vi "Auto.vi"() -> ()   [LabVIEW 2020]
uses:
  Global_Variable/Global.vi
  Global_Variable/A180648.vi
  Global_Variable/System_Conf.vi
  Libraries/S7/S7.lvlib
panel:
  out "前序":string
  out "用户事件输出":refnum<user-event>
  out "磨合正向初始化":bool
  out "工位三开始计时1":bool
  out "产品变更_Event":refnum<user-event>
  out "T1+T2":dbl
  out "T2":dbl
  out "T1":dbl
  out "吸收电流":sgl
  out "输出扭矩(大)":sgl
  out "输入扭矩":sgl
  out "力特性逆向去程":bool
  out "力特性正向去程":bool
  out "力特性逆向回程":bool
  out "力特性正向回程":bool
  out "工位三开始计时":bool
  out "工位二开始计时":bool
  out "功能正向初始化":bool
  out "功能逆向初始化":bool
  out "空载逆向初始化":bool
  out "空载正向初始化":bool
  out "试验项目":T1(tab)
  out "拉压曲线":cluster{dbl[], dbl[]}[](graph)
  out "侧铆曲线":cluster{dbl[], dbl[]}[](graph)
  out "0°曲线":cluster{dbl[], dbl[]}[](graph)
  out "45°曲线":cluster{dbl[], dbl[]}[](graph)
  out "力特性试验":cluster{dbl[], dbl[]}[](graph)
  out "功能试验":cluster{dbl[], dbl[]}[](graph)
  out "电流特性试验":cluster{dbl[], dbl[]}[](graph)
  out "逆向空载试验":cluster{dbl[], dbl[]}[](graph)
  out "磨合":cluster{dbl[], dbl[]}[](graph)
  in  "判定结果":bool[][](array[boolean])=[[TRUE]]
  in  "STEP":string
  # "车速0"
  # "车速1"
  # "车速2"
  # "车速3"
  # "车速4"
  # "车速5"
  # "车速0"
  # "车速1"
  # "车速2"
  # "车速3"
  # "车速4"
  # "车速5"
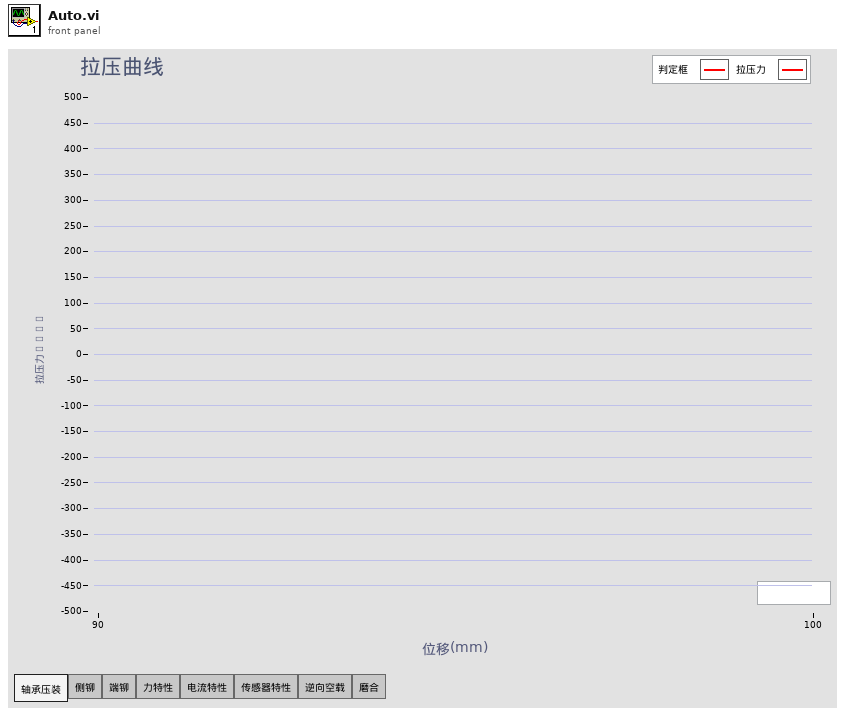
[diagram p1: front panel]
types:
  T1 = enum32{"轴承压装", "侧铆", "端铆", "力特性", "电流特性", "传感器特性", "逆向空载", "磨合"}
  T2 = enum32{"Invalid", "Standard", "Closed", "Hidden", "Minimized", "Maximized"}
  T3 = cluster{"输入轴扭矩":dbl, "输出轴扭矩小量程":dbl, "输出轴扭矩大量程":dbl}
  T4 = typedef "System_conf.ctl" = cluster{"空载滤波":bool, "逆向空载滤波":bool, "空载扭矩系数":dbl, "逆向空载扭矩系数":dbl}
  T5 = cluster{"位移":cluster{"单位":string, "下限":dbl, "上限":dbl}, "拉力":cluster{"单位":string, "下限":dbl, "上限":dbl}, "位移1":cluster{"单位":string, "下限":dbl, "上限":dbl}, "压力":cluster{"单位":string, "下限":dbl, "上限":dbl}}
  T6 = cluster{"拉力最大值":cluster{"单位":string, "下限":dbl, "上限":dbl}, "拉力最小值":cluster{"单位":string, "下限":dbl, "上限":dbl}, "拉力波动":cluster{"单位":string, "下限":dbl, "上限":dbl}, "压力最大值":cluster{"单位":string, "下限":dbl, "上限":dbl}, "压力最小值":cluster{"单位":string, "下限":dbl, "上限":dbl}, "压力波动":cluster{"单位":string, "下限":dbl, "上限":dbl}}
  T7 = cluster{"输入旋转位移":sgl, "电缸":sgl, "工装移载位移":sgl, "345":sgl, "电缸位移":sgl, "打算":sgl, "输出扭矩(大)":sgl, "132":sgl, "拉压力":sgl, "sad":sgl}
  T8 = typedef "lveventtype.ctl" = enum32{"Null", "Timeout", "Annotation Menu Selection", "Annotation Menu Selection?", "App Instance Close", "App Instance Close?", "Autoscale Range Change", "Bookmark Info Change", "Cell Edit", "Cell Edit?", "Cursor Grab", "Cursor Grab?", "Cursor Menu Selection", "Cursor Menu Selection?", "Cursor Move", "Cursor Release", "Data Change", "Direction Change", "Display State Change", "Drag Ended", "Drag Enter", "Drag Leave", "Drag Over", "Drag Source Update", "Drag Starting", "Drag Starting?", "Drop", "Exec State Change", "Key Down", "Key Down?", "Key Repeat", "Key Repeat?", "Key Up", "Listbox Double Click", "Menu Activation?", "Menu Selection (App)", "Menu Selection? (App)", "Menu Selection (User)", "Mouse Down", "Mouse Down?", "Mouse Enter", "Mouse Leave", "Mouse Move", "Mouse Up", "Mouse Wheel", "NI Security User Change (App)", "Pane Size", "Panel Close", "Panel Close?", "Panel Resize", "Plot Attribute Change", "Scale Range Change", "Shortcut Menu Activation?", "Shortcut Menu Selection (App)", "Shortcut Menu Selection? (App)", "Shortcut Menu Selection (User)", "Tree Double Click", "Tree Drag", "Tree Drag?", "Tree Drop", "Tree Drop?", "Tree Item Close", "Tree Item Close?", "Tree Item Open", "Tree Item Open?", "User Event", "Value Change"}
  T9 = typedef "LVPoint32TypeDef.ctl" = cluster{"Horizontal":i32, "Vertical":i32}
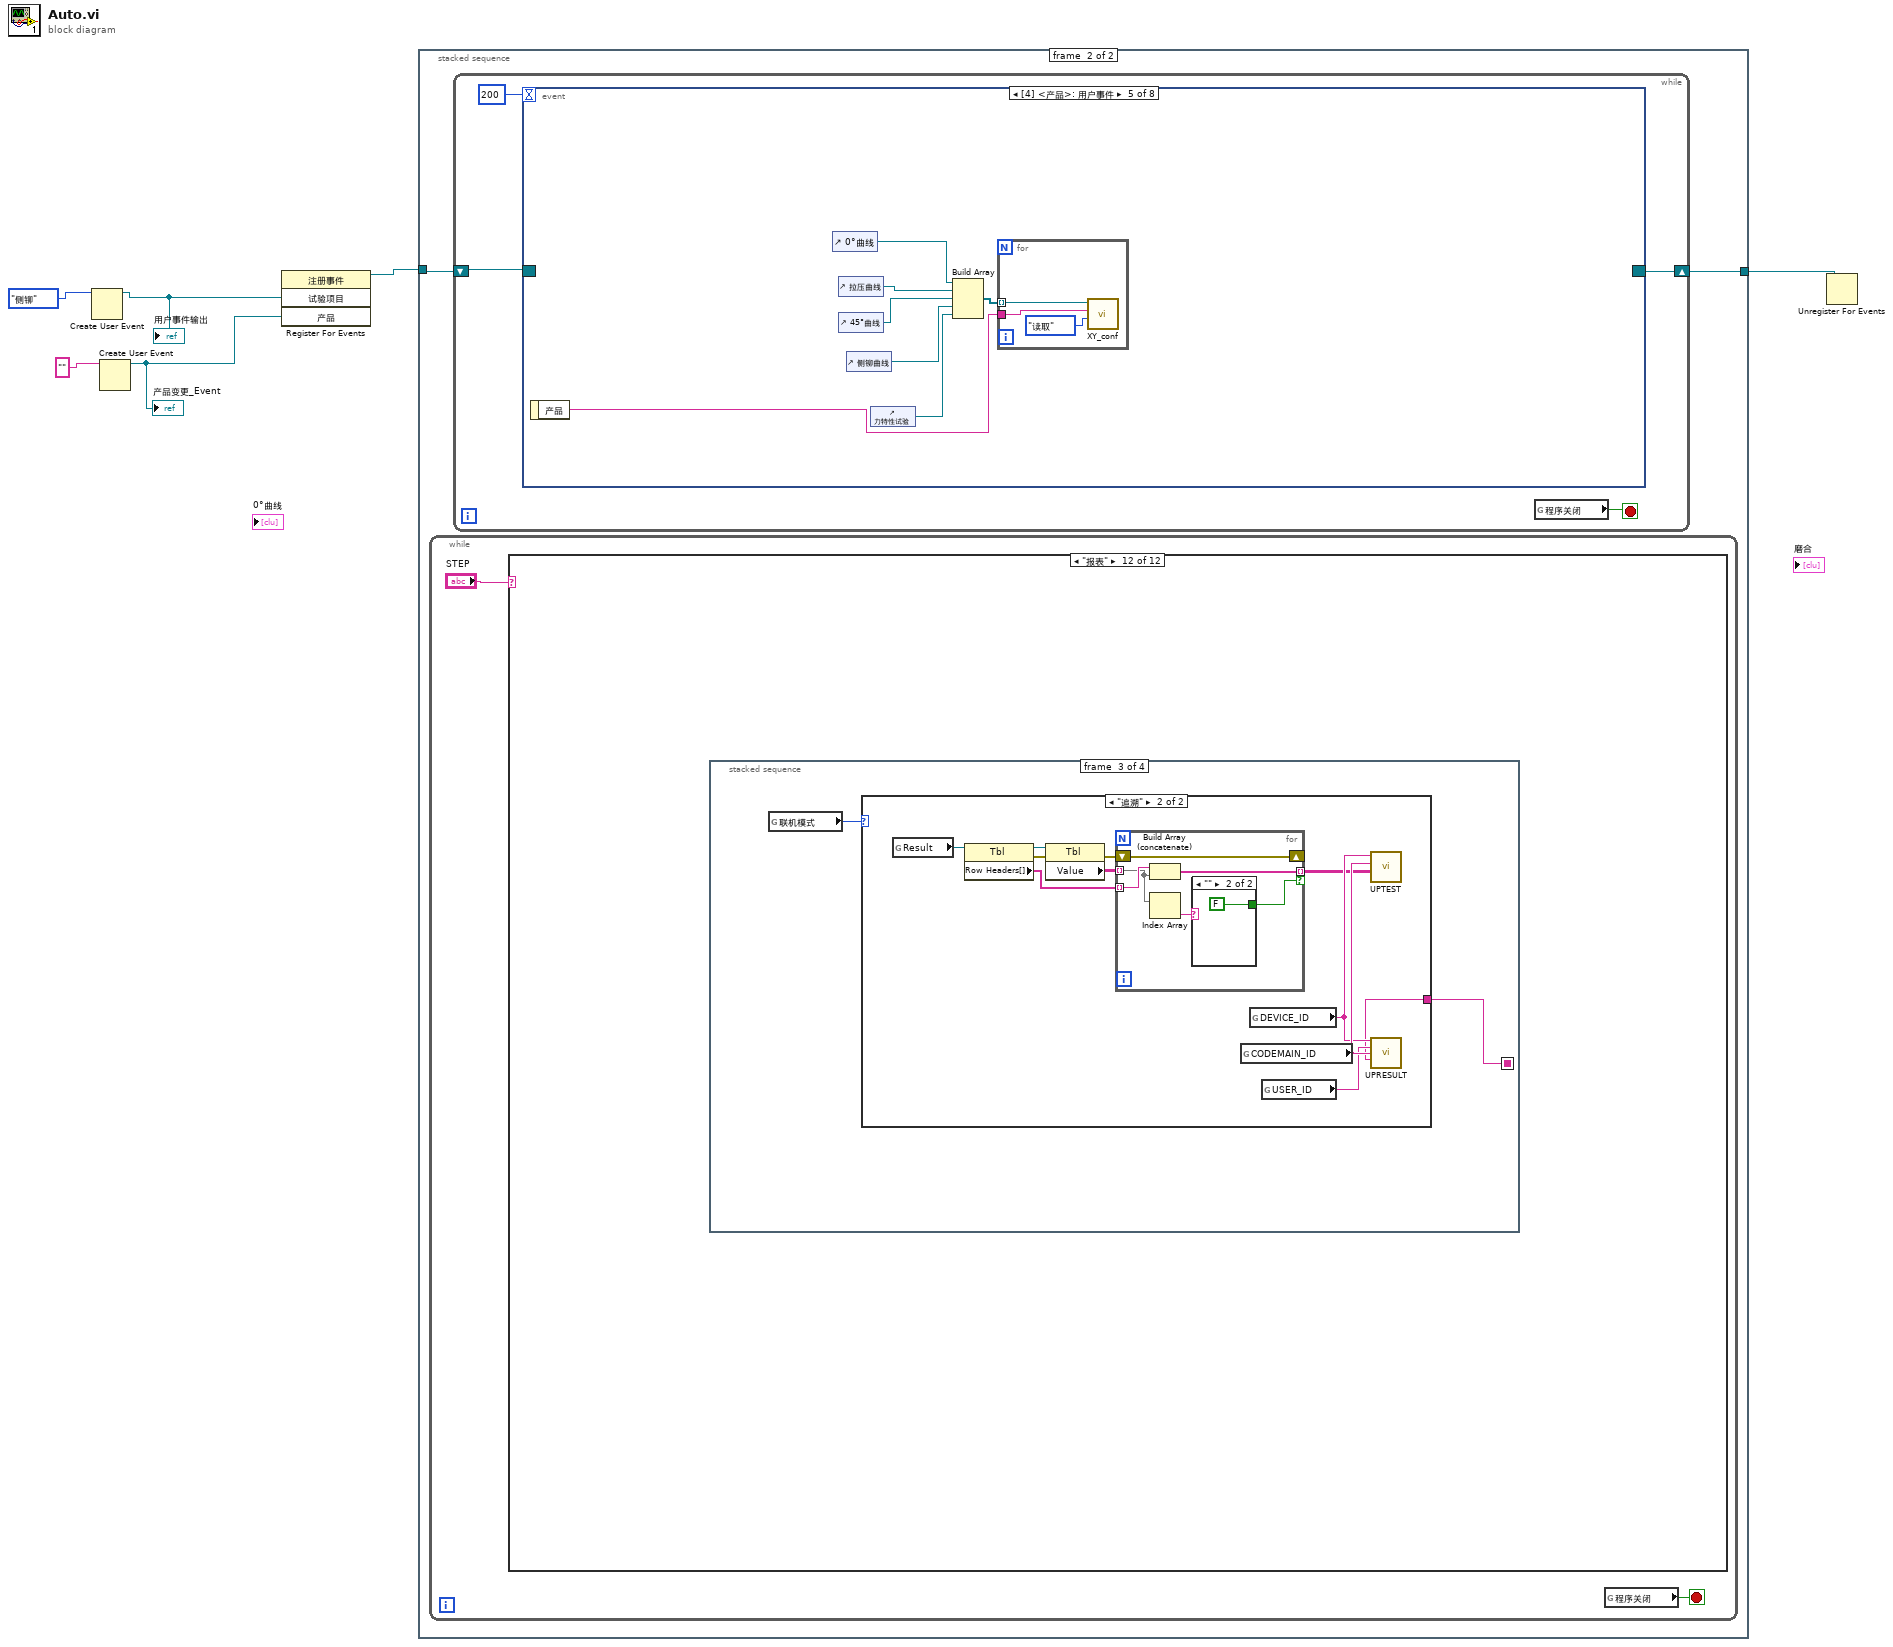
[diagram p0: block diagram]
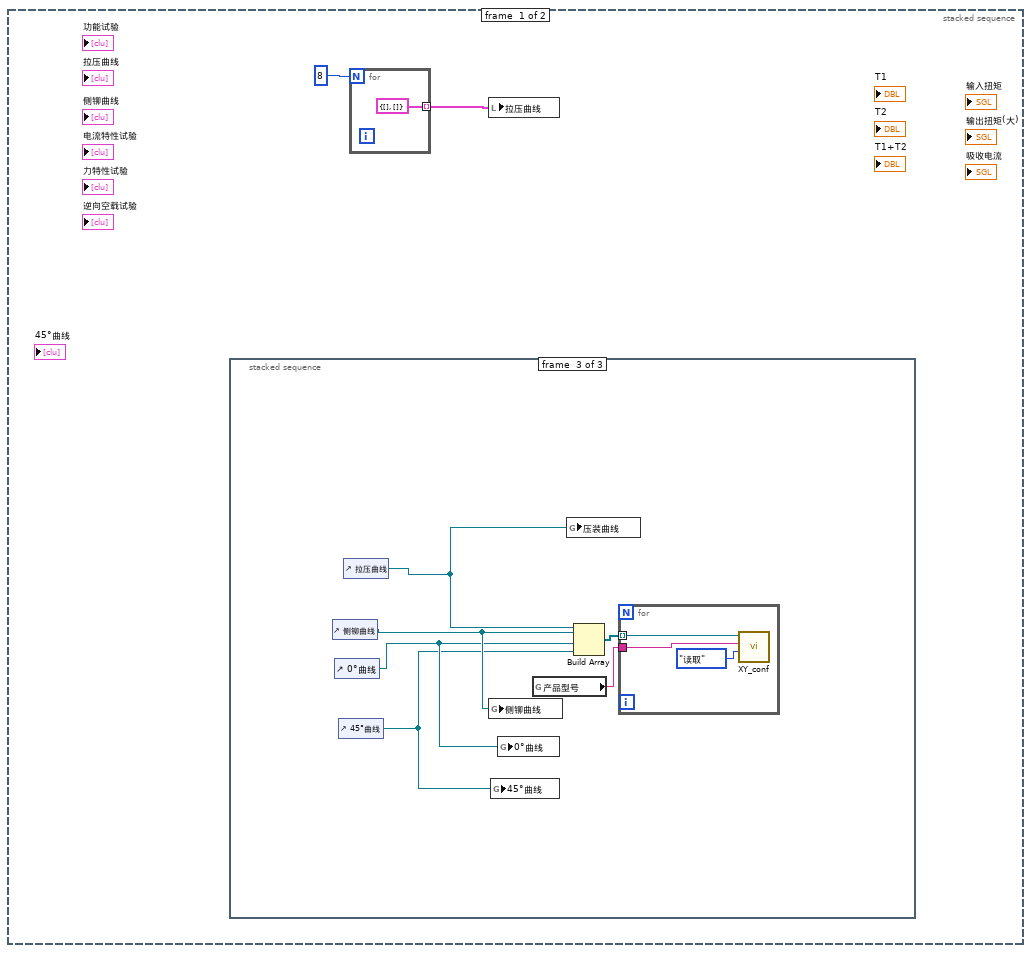
[diagram p2: hidden frame]
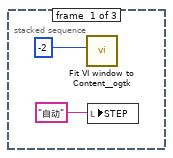
[diagram p3: hidden frame]
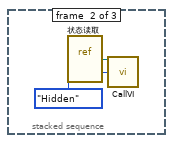
[diagram p4: hidden frame]
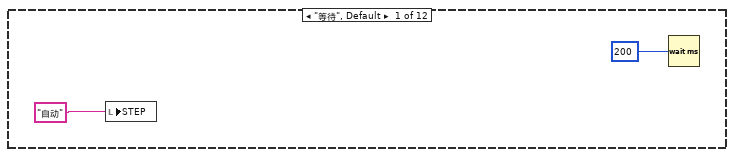
[diagram p5: hidden frame]
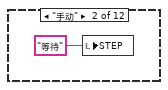
[diagram p6: hidden frame]
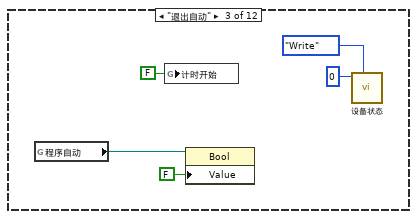
[diagram p7: hidden frame]
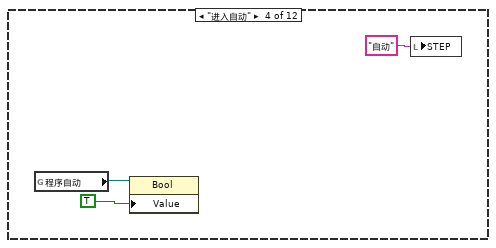
[diagram p8: hidden frame]
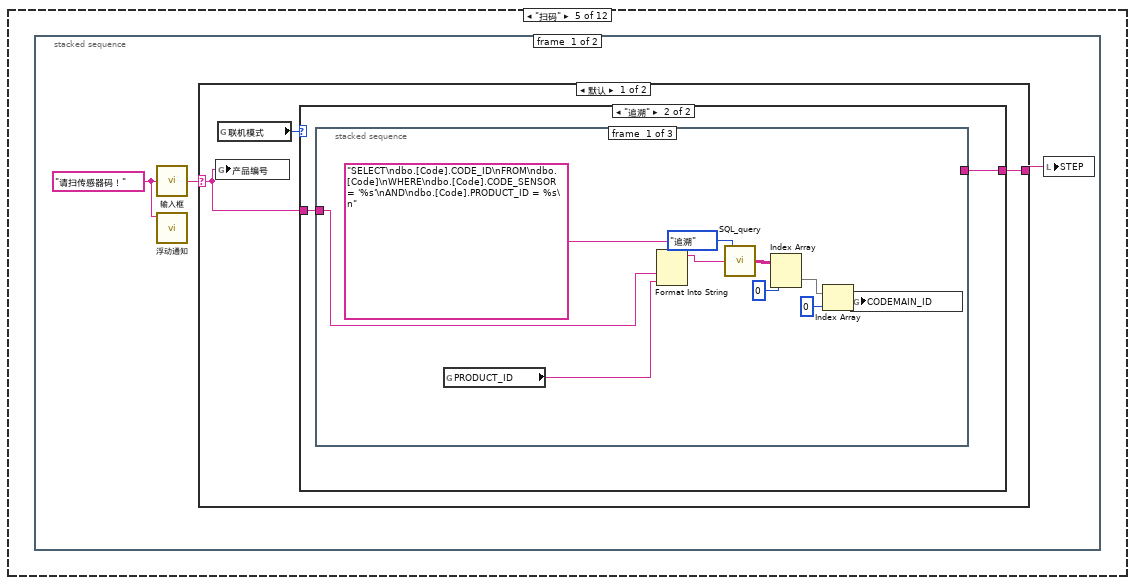
[diagram p9: hidden frame]
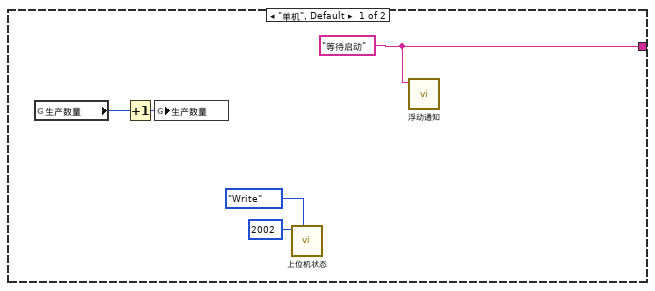
[diagram p10: hidden frame]
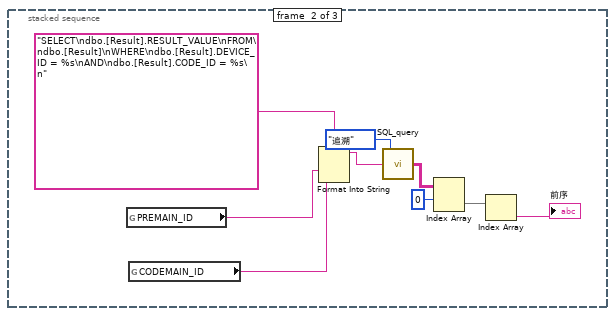
[diagram p11: hidden frame]
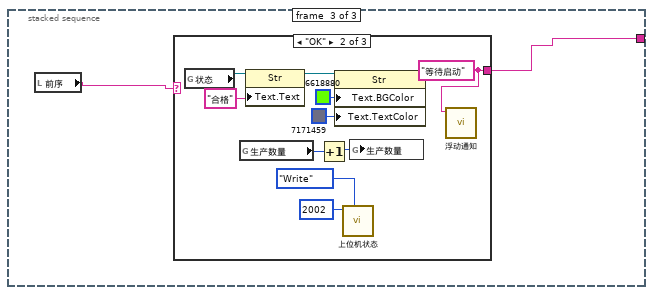
[diagram p12: hidden frame]
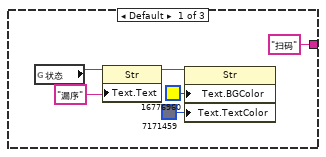
[diagram p13: hidden frame]
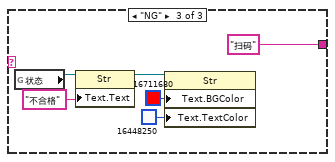
[diagram p14: hidden frame]
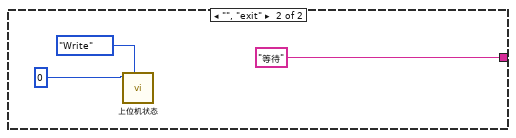
[diagram p15: hidden frame]
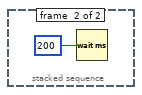
[diagram p16: hidden frame]
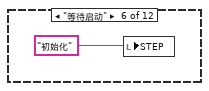
[diagram p17: hidden frame]
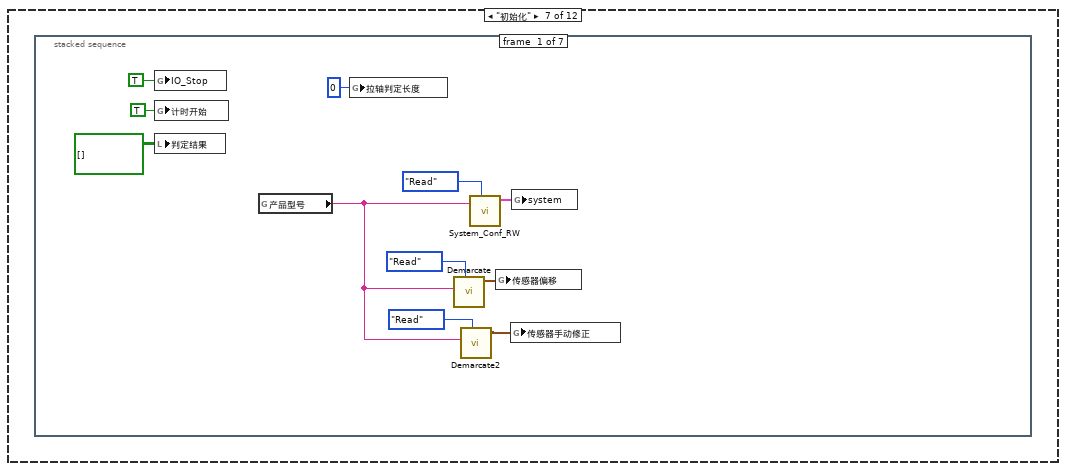
[diagram p18: hidden frame]
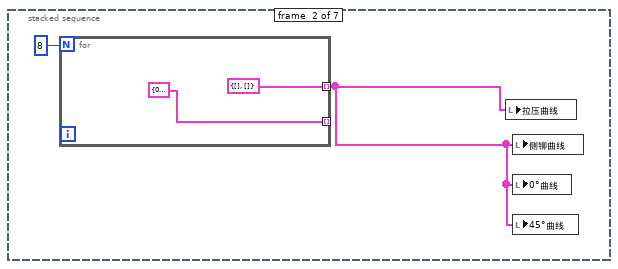
[diagram p19: hidden frame]
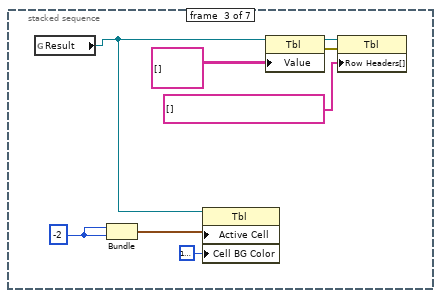
[diagram p20: hidden frame]
diagram:
  n1 = Create User Event(user event datatype=T1."侧铆" ("试验项目")) -> (user event=w1:refnum<user-event>)  [unwired: 1 in, 1 out]
  "用户事件输出" <- w1
  n2 = Create User Event(user event datatype="" ("产品")) -> (user event=w3:refnum<user-event>)  [unwired: 1 in, 1 out]
  "产品变更_Event" <- w3
  n3 = register-events(w1, w3) -> (reference out=w6:refnum<event-registration>)  [unwired: 2 in, 1 out]
  n4 = stacked-sequence {
    tunnel: w6 -> [_ w24]
    tunnel: [_ w23] -> w5
    frame #0 {
      n5 = stacked-sequence {
        frame #0 {
          n6 = call <userlib>:"Fit VI window to Content__ogtk.vi"("border spacing (2 px)"=-2) -> ()  [unwired: 5 in, 2 out]
          n7 = local write "STEP"("自动" ("STEP")) -> ()
        }
        frame #1 {
          n8 = vi-ref "状态读取.vi"() -> (w13:refnum<vi>)
          n9 = call "CallVI.vi"("VI引用"=w13, "状态"=T2."Hidden") -> ()  [unwired: 12 in, 2 out]
        }
        frame #2 {
          n10 = control-ref of="侧铆曲线"() -> (w17:refnum<vi>)
          n11 = control-ref of="0°曲线"() -> (w16:refnum<vi>)
          n12 = control-ref of="45°曲线"() -> (w15:refnum<vi>)
          n13 = control-ref of="拉压曲线"() -> (w14:refnum<vi>)
          n14 = global write "A180648.vi" "侧铆曲线"(w17) -> ()
          n15 = global write "A180648.vi" "45°曲线"(w15) -> ()
          n16 = global write "A180648.vi" "0°曲线"(w16) -> ()
          n17 = global read "Global.vi" "产品型号"() -> (w18:string)
          n18 = global write "A180648.vi" "压装曲线"(w14) -> ()
          n19 = Build Array(w14, w17, w16, w15) -> (w19:refnum<vi>[])
          n20 = for {
            tunnel: w19 -> [w21] mode=indexing
            tunnel: w18 -> [w20]
            n21 = call "XY_conf.vi"("方式"=enum16{"写入", "读取"}."读取", "产品"=w20, "XY图引用"=w21) -> ()  [unwired: 4 in, 1 out]
          }
        }
      }
      n22 = for {
        N: 8 -> [_]
        tunnel: [cluster{dbl[], dbl[]} {[], []}] -> w8 mode=indexing
      }
      n23 = local write "拉压曲线"(w8) -> ()
    }
    frame #1 {
      n24 = while {
        stop <- w26 stop-if-true
        n25 = case shown="\"报表\"" "STEP" {
          frame "等待", Default {
            n26 = local write "STEP"("自动" ("STEP")) -> ()
            n27 = Wait (ms)(milliseconds to wait=u32 200 ("等待时间（毫秒）")) -> ()  [unwired: 1 out]
          }
          frame "手动" {
            n28 = local write "STEP"("等待" ("STEP")) -> ()
          }
          frame "退出自动" {
            n29 = global read "Global.vi" "程序自动"() -> (w31:refnum<vi>)
            n30 = global write "Global.vi" "计时开始"(FALSE ("计时开始")) -> ()
            n31 = property class="Bool"(reference=w31, "Value"=FALSE) -> ()  [unwired: 1 in, 2 out]
            n32 = call "设备状态.vi"("枚举"=enum16{"Read", "Write"}."Write", "Status_Write"=i16 0) -> ()  [unwired: 9 in, 1 out]
          }
          frame "进入自动" {
            n33 = global read "Global.vi" "程序自动"() -> (w36:refnum<vi>)
            n34 = property class="Bool"(reference=w36, "Value"=TRUE) -> ()  [unwired: 1 in, 2 out]
            n35 = local write "STEP"("自动" ("STEP")) -> ()
          }
          frame "扫码" {
            n36 = stacked-sequence {
              frame #0 {
                w39 = "请扫传感器码！" ("提示信息")
                n37 = call "输入框.vi"("提示信息"=w39) -> ("条形码输出"=w40:string)
                n38 = call "浮动通知.vi"("通知内容"=w39) -> ()  [unwired: 11 in]
                n39 = case shown="默认" w40 {
                  selector: w40 -> [w41 _]
                  tunnel: [w43 "等待" ("State(s) in Front (\"\")")] -> w38
                  frame Default {
                    n40 = global write "Global.vi" "产品编号"(w41) -> ()
                    n41 = global read "Global.vi" "联机模式"() -> (w42:enum16{"单机", "追溯"})
                    n42 = case shown="\"追溯\"" w42 {
                      tunnel: [w46 w50] -> w43
                      tunnel: w41 -> [_ w49]
                      frame "单机", Default {
                        w46 = "等待启动" ("State(s) in Front (\"\")")
                        n43 = global read "Global.vi" "生产数量"() -> (w47:i32)
                        n44 = Increment(x=w47) -> (x+1=w48:i32)
                        n45 = global write "Global.vi" "生产数量"(w48) -> ()
                        n46 = call "上位机状态.vi"("枚举"=enum16{"Read", "Write"}."Write", "Status_Write"=i16 2002) -> ()  [unwired: 9 in, 1 out]
                        n47 = call "浮动通知.vi"("通知内容"=w46) -> ()  [unwired: 11 in]
                      }
                      frame "追溯" {
                        n48 = stacked-sequence {
                          tunnel: [_ _ w71] -> w50
                          tunnel: w49 -> [w59 _ _]
                          frame #0 {
                            n49 = global read "追溯Global.vi" "PRODUCT_ID"() -> (w58:string)
                            n50 = Format Into String(format string="SELECT\ndbo.[Code].CODE_ID\nFROM\ndbo.[Code]\nWHERE\ndbo.[Code].CODE_SENSOR = '%s'\nAND\ndbo.[Code].PRODUCT_ID = %s\n" ("格式字符串"), w59, w58) -> (resulting string=w57:string)  [unwired: 2 in, 1 out]
                            n51 = call "SQL_query.vi"("SQL query"=w57, "联机模式"=enum16{"单机", "追溯"}."追溯") -> ("data"=w55:string[][])  [unwired: 2 in, 1 out]
                            n52 = Index Array(array=w55, index (row)=0 ("索引 (行)")) -> (element=w53:string[])  [unwired: 1 in]
                            n53 = Index Array(array=w53, index=0 ("索引")) -> (element=w51:string)
                            n54 = global write "追溯Global.vi" "CODEMAIN_ID"(w51) -> ()
                          }
                          frame #1 {
                            n55 = global read "追溯Global.vi" "PREMAIN_ID"() -> (w68:string)
                            n56 = global read "追溯Global.vi" "CODEMAIN_ID"() -> (w67:string)
                            n57 = Format Into String(format string="SELECT\ndbo.[Result].RESULT_VALUE\nFROM\ndbo.[Result]\nWHERE\ndbo.[Result].DEVICE_ID = %s\nAND\ndbo.[Result].CODE_ID = %s\n" ("格式字符串"), w68, w67) -> (resulting string=w66:string)  [unwired: 2 in, 1 out]
                            n58 = call "SQL_query.vi"("SQL query"=w66, "联机模式"=enum16{"单机", "追溯"}."追溯") -> ("data"=w64:string[][])  [unwired: 2 in, 1 out]
                            n59 = Index Array(array=w64, index (row)=0 ("索引 (行)")) -> (element=w62:string[])  [unwired: 1 in]
                            n60 = Index Array(array=w62) -> (element=→"前序":string)  [unwired: 1 in]
                          }
                          frame #2 {
                            n61 = local read "前序"() -> (w70:string)
                            n62 = case shown="\"OK\"" w70 {
                              tunnel: ["扫码" ("State(s) in Front (\"\")") w82 "扫码" ("State(s) in Front (\"\")")] -> w71
                              frame Default {
                                n63 = global read "Global.vi" "状态"() -> (w77:refnum<vi>)
                                n64 = property class="Str"(reference=w77, "Text.Text"="漏序" ("文本.文本")) -> (reference out=w76:refnum<vi>)  [unwired: 1 in, 1 out]
                                n65 = property class="Str"(reference=w76, "Text.BGColor"=u32 16776960 ("文本.文本颜色:背景色"), "Text.TextColor"=u32 7171459 ("文本.文本颜色:文本颜色")) -> ()  [unwired: 1 in, 2 out]
                              }
                              frame "OK" {
                                w82 = "等待启动" ("State(s) in Front (\"\")")
                                n66 = global read "Global.vi" "状态"() -> (w87:refnum<vi>)
                                n67 = global read "Global.vi" "生产数量"() -> (w80:i32)
                                n68 = property class="Str"(reference=w87, "Text.Text"="合格" ("文本.文本")) -> (reference out=w85:refnum<vi>)  [unwired: 1 in, 1 out]
                                n69 = Increment(x=w80) -> (x+1=w81:i32)
                                n70 = property class="Str"(reference=w85, "Text.BGColor"=u32 6618880 ("文本.文本颜色:背景色"), "Text.TextColor"=u32 7171459 ("文本.文本颜色:文本颜色")) -> ()  [unwired: 1 in, 2 out]
                                n71 = call "上位机状态.vi"("枚举"=enum16{"Read", "Write"}."Write", "Status_Write"=i16 2002) -> ()  [unwired: 9 in, 1 out]
                                n72 = global write "Global.vi" "生产数量"(w81) -> ()
                                n73 = call "浮动通知.vi"("通知内容"=w82) -> ()  [unwired: 11 in]
                              }
                              frame "NG" {
                                n74 = global read "Global.vi" "状态"() -> (w93:refnum<vi>)
                                n75 = property class="Str"(reference=w93, "Text.Text"="不合格" ("文本.文本")) -> (reference out=w91:refnum<vi>)  [unwired: 1 in, 1 out]
                                n76 = property class="Str"(reference=w91, "Text.BGColor"=u32 16711680 ("文本.文本颜色:背景色"), "Text.TextColor"=u32 16448250 ("文本.文本颜色:文本颜色")) -> ()  [unwired: 1 in, 2 out]
                              }
                            }
                          }
                        }
                      }
                    }
                  }
                  frame "", "exit" {
                    n77 = call "上位机状态.vi"("枚举"=enum16{"Read", "Write"}."Write", "Status_Write"=u16 0 ("设备状态")) -> ()  [unwired: 9 in, 1 out]
                  }
                }
                n78 = local write "STEP"(w38) -> ()
              }
              frame #1 {
                n79 = Wait (ms)(milliseconds to wait=u32 200 ("等待时间（毫秒）")) -> ()  [unwired: 1 out]
              }
            }
          }
          frame "等待启动" {
            n80 = local write "STEP"("初始化" ("STEP")) -> ()
          }
          frame "初始化" {
            n81 = stacked-sequence {
              frame #0 {
                n82 = global write "Global.vi" "IO_Stop"(TRUE ("IO_Stop")) -> ()
                n83 = global write "Global.vi" "计时开始"(TRUE ("计时开始")) -> ()
                n84 = local write "判定结果"(bool[][] [] ("判定结果")) -> ()
                n85 = global read "Global.vi" "产品型号"() -> (w100:string)
                n86 = global write "判定参数.vi" "拉轴判定长度"(0 ("拉轴判定长度")) -> ()
                n87 = call "Demarcate.vi"("Mode"=enum16{"Read", "Write"}."Read", "Section"=w100) -> ("Sensor OUT"=w104:T3)  [unwired: 8 in, 1 out]
                n88 = call "Demarcate2.vi"("Mode"=enum16{"Read", "Write"}."Read", "Section"=w100) -> ("Sensor OUT"=w103:T3)  [unwired: 8 in, 1 out]
                n89 = call "System_Conf_RW.vi"("Mode"=enum16{"Read", "Write"}."Read", "Section"=w100) -> ("system_out"=w106:T4)  [unwired: 8 in, 1 out]
                n90 = global write "传感器偏移.vi" "传感器偏移"(w104) -> ()
                n91 = global write "传感器偏移.vi" "传感器手动修正"(w103) -> ()
                n92 = global write "System_Conf.vi" "system"(w106) -> ()
              }
              frame #1 {
                n93 = for {
                  N: 8 -> [_]
                  tunnel: [cluster{dbl[], dbl[]} {[], []}] -> w110 mode=indexing
                  tunnel: [cluster{"f0":dbl, "df":dbl, "magnitude":dbl[]} {"f0"=0.0, "df"=0.0, "magnitude"=[]} ("power spectrum [dB EU]")] -> _ mode=indexing
                }
                n94 = local write "拉压曲线"(w110) -> ()
                n95 = local write "侧铆曲线"(w110) -> ()
                n96 = local write "0°曲线"(w110) -> ()
                n97 = local write "45°曲线"(w110) -> ()
              }
              frame #2 {
                w115 = -2
                n98 = global read "Global.vi" "Result"() -> (w117:refnum<vi>)
                n99 = Bundle(w115, w115) -> (w114:cluster{i32, i32})  [unwired: 1 in]
                n100 = property class="Tbl"(reference=w117, "Active Cell"=w114, "Cell BG Color"=u32 16777216 ("活动单元格:单元格背景色")) -> ()  [unwired: 1 in, 2 out]
                n101 = property class="Tbl"(reference=w117, "Value"=string[][] []) -> (reference out=w120:refnum<vi>, error out=w121:errorcluster)  [unwired: 1 in]
                n102 = property class="Tbl"(reference=w120, error in=w121, "Row Headers[]"=string[] [] ("列首字符串[]")) -> ()  [unwired: 2 out]
              }
              frame #3 {
                n103 = global read "A180648.vi" "LED-轴承压装"() -> (w125:refnum<vi>)
                n104 = global read "A180648.vi" "LED-端铆"() -> (w122:refnum<vi>)
                n105 = global read "A180648.vi" "LED-侧铆"() -> (w123:refnum<vi>)
                n106 = Build Array(w125, w123, w122) -> (w124:refnum<vi>[])
                n107 = for {
                  tunnel: w124 -> [w126] mode=indexing
                  n108 = property class="Bool"(reference=w126, "Colors [4]"=cluster{u32, u32}[] [{12369084, 12369084}] ("颜色[4]")) -> ()  [unwired: 1 in, 2 out]
                }
              }
              frame #4 {
                w129 = 1 ("维数大小")
                n109 = Initialize Array(" " ("字符串"), w129, w129, w129) -> (w131:string[][][])
                n110 = global write "A180648.vi" "当前检测项"(enum32{"拉轴", "卡簧", "完成"}."拉轴" ("当前检测项")) -> ()
                n111 = global write "A180648.vi" "检测结果"(w131) -> ()
              }
              frame #5 {
                n112 = local read "拉压曲线"() -> (w133:cluster{dbl[], dbl[]}[])
                n113 = global read "判定参数.vi" "判定框"() -> (w134:T5)
                n114 = for {
                  tunnel: w133 -> [w137] mode=indexing
                  tunnel: [w136] -> w132 mode=indexing
                  tunnel: w134 -> [w135]
                  i -> [w138]
                  n115 = case shown="1" w138 {
                    tunnel: w137 -> [w139 _ _]
                    tunnel: [w139 w142 w152] -> w136
                    tunnel: w135 -> [_ w147 w157]
                    frame Default {
                    }
                    frame 0 {
                      n116 = Unbundle By Name(w147) -> ("位移.下限"=w146:dbl, "位移.上限"=w145:dbl, "压力.下限"=w140:dbl, "压力.上限"=w141:dbl)
                      n117 = Build Array(w145, w145, w146, w146, w145) -> (w144:dbl[])
                      n118 = Build Array(w140, w141, w141, w140, w140) -> (w143:dbl[])
                      n119 = Bundle(w144, w143) -> (w142:cluster{dbl[], dbl[]})  [unwired: 1 in]
                    }
                    frame 1 {
                      n120 = Unbundle By Name(w157) -> ("位移.下限"=w156:dbl, "位移.上限"=w155:dbl, "压力.上限"=w150:dbl, "压力.下限"=w151:dbl)
                      n121 = Negate(x=w150) -> (-x=w149:dbl)
                      n122 = Negate(x=w151) -> (-x=w148:dbl)
                      n123 = Build Array(w155, w155, w156, w156, w155) -> (w154:dbl[])
                      n124 = Build Array(w149, w148, w148, w149, w149) -> (w153:dbl[])
                      n125 = Bundle(w154, w153) -> (w152:cluster{dbl[], dbl[]})  [unwired: 1 in]
                    }
                  }
                }
                n126 = local write "拉压曲线"(w132) -> ()
              }
              frame #6 {
                w159 = TRUE
                n127 = local write "STEP"("自动" ("STEP")) -> ()
                "工位三开始计时" <- w159
                "工位二开始计时" <- w159
                "空载正向初始化" <- w159
                "空载逆向初始化" <- w159
                "功能正向初始化" <- w159
                "功能逆向初始化" <- w159
                "力特性逆向去程" <- w159
                "力特性正向去程" <- w159
                "力特性逆向回程" <- w159
                "力特性正向回程" <- w159
                "磨合正向初始化" <- w159
                "工位三开始计时1" <- w159
              }
            }
          }
          frame "试验项" {
            n128 = global read "A180648.vi" "当前检测项"() -> (w160:enum32{"拉轴", "卡簧", "完成"})
            n129 = case shown="\"拉轴\", 默认" w160 {
              selector: w160 -> [w162 _]
              tunnel: [w165 "报表" ("STEP")] -> w161
              frame "拉轴", Default {
                n130 = global read "Global.vi" "试验项目"() -> (w163:bool[])
                n131 = Index Array(array=w163, index=w162) -> (element=w164:bool)
                n132 = case shown="假" w164 {
                  tunnel: ["试验项" ("字符串") w172] -> w165
                  tunnel: w162 -> [_ w173]
                  frame False {
                    n133 = global read "A180648.vi" "当前检测项"() -> (w170:enum32{"拉轴", "卡簧", "完成"})
                    n134 = Increment(x=w170) -> (x+1=w169:enum32{"拉轴", "卡簧", "完成"})
                    n135 = global write "A180648.vi" "当前检测项"(w169) -> ()
                    n136 = local read "判定结果"() -> (w166:bool[][])
                    n137 = Build Array (concatenate)(w166, bool[] [FALSE] ("判定结果")) -> (w167:bool[][])
                    n138 = local write "判定结果"(w167) -> ()
                  }
                  frame True {
                    n139 = case shown="\"卡簧\"" w173 {
                      tunnel: ["等待" ("STEP") "等待" ("STEP") "报表" ("STEP")] -> w172
                      frame "拉轴", Default {
                        n140 = call "浮动通知.vi"("通知内容"="拉拔力试验") -> ()  [unwired: 11 in]
                        n141 = property on="试验项目" class="TabCtl (严格)"("Val(Sgnl)"=T1."轴承压装" ("值(信号)")) -> ()  [unwired: 2 in, 2 out]
                      }
                      frame "卡簧" {
                        n142 = call "浮动通知.vi"("通知内容"="卡簧检测") -> ()  [unwired: 11 in]
                      }
                      frame "完成" {
                      }
                    }
                  }
                }
              }
              frame "完成" {
              }
            }
            n143 = local write "STEP"(w161) -> ()
          }
          frame "判定" {
            n144 = stacked-sequence {
              frame #0 {
                n145 = call "备用1.vi"("枚举"=enum16{"Read", "Write"}."Write", "Status_Write"=i16 0) -> ()  [unwired: 9 in, 1 out]
              }
              frame #1 {
                n146 = global read "判定参数.vi" "拉压判定参数"() -> (w194:T6)
                n147 = local read "拉压曲线"() -> (w195:cluster{dbl[], dbl[]}[])
                n148 = global read "Global.vi" "Result"() -> (w193:refnum<vi>)
                n149 = call "压装试验判定.vi"("Result"=w193, "判定参数"=w194, "XY曲线"=w195) -> ("判定项长度"=w184:i32, "OK？"=w183:bool)  [unwired: 7 in]
                n150 = global read "A180648.vi" "LED-轴承压装"() -> (w189:refnum<vi>)
                n151 = local read "判定结果"() -> (w185:bool[][])
                n152 = Select(t=cluster{u32, u32}[] [{6618880, 6618880}, {6618880, 6618880}, {6618880, 6618880}, {6618880, 6618880}] ("颜色[4]"), s=w183, f=cluster{u32, u32}[] [{16711680, 16711680}, {16711680, 16711680}, {16711680, 16711680}, {16711680, 16711680}] ("颜色[4]")) -> (s? t:f=w190:cluster{u32, u32}[])
                n153 = Build Array(TRUE, w183) -> (w188:bool[])
                n154 = global write "判定参数.vi" "拉轴判定长度"(w184) -> ()
                n155 = property class="Bool"(reference=w189, "Colors [4]"=w190) -> ()  [unwired: 1 in, 2 out]
                n156 = Build Array (concatenate)(w185, w188) -> (w186:bool[][])
                n157 = case shown="假" w183 {
                  frame False {
                    n158 = call "备用2.vi"("枚举"=enum16{"Read", "Write"}."Write", "Status_Write"=u16 2 ("工位1合格状态")) -> ()  [unwired: 9 in, 1 out]
                  }
                  frame True {
                    n159 = call "备用2.vi"("枚举"=enum16{"Read", "Write"}."Write", "Status_Write"=u16 1 ("工位1合格状态")) -> ()  [unwired: 9 in, 1 out]
                  }
                }
                n160 = local write "判定结果"(w186) -> ()
              }
              frame #2 {
                n161 = local write "STEP"("报表") -> ()
              }
            }
          }
          frame "自动" {
            n162 = global read "Global.vi" "复测状态"() -> (w202:i16)
            n163 = case shown="56" w202 {
              frame -128 {
                n164 = global write "Global.vi" "计时开始"(FALSE ("计时开始")) -> ()
                n165 = call "浮动通知.vi"("通知内容"="复位中……" ("Status")) -> ()  [unwired: 11 in]
              }
              frame Default {
              }
              frame 0 {
                n166 = disable-structure shown="禁用" {
                  frame Disabled {
                    n167 = global write "Global.vi" "计时开始"(FALSE ("计时开始")) -> ()
                  }
                  frame Enabled {
                  }
                }
              }
              frame 1 {
                n168 = disable-structure shown="禁用" {
                  frame Disabled {
                    n169 = local read "拉压曲线"() -> (w244:cluster{dbl[], dbl[]}[])
                    n170 = for {
                      tunnel: [w246] -> _ mode=indexing
                      tunnel: w244 -> [w245] mode=indexing
                      i -> [w247]
                      n171 = case shown="2" w247 {
                        tunnel: [_ w248] -> w246
                        tunnel: w245 -> [_ w253]
                        frame Default {
                        }
                        frame 2 {
                          n172 = Unbundle(w253) -> (w252:dbl[], w251:dbl[])
                          n173 = Build Array(w252) -> (w250:dbl[][])  [unwired: 1 in]
                          n174 = Build Array(w251) -> (w249:dbl[][])  [unwired: 1 in]
                          n175 = Bundle(w250, w249) -> (w248:cluster{dbl[][], dbl[][]})  [unwired: 1 in]
                        }
                      }
                    }
                    n176 = local read "拉压曲线"() -> ()  [unwired: 1 in]
                  }
                  frame Enabled {
                  }
                }
              }
              frame 2 {
              }
              frame 8 {
                n177 = call "浮动通知.vi"("通知内容"="程序停止！" ("Status")) -> ()  [unwired: 11 in]
              }
              frame 10 {
              }
              frame 20 {
              }
              frame 51 {
                n178 = call "浮动通知.vi"("通知内容"="请锁紧手柄并点击确定" ("Status")) -> ()  [unwired: 11 in]
              }
              frame 52 {
                n179 = call "浮动通知.vi"("通知内容"="请启动" ("Status")) -> ()  [unwired: 11 in]
              }
              frame 54 {
                n180 = call "浮动通知.vi"("通知内容"="等待到达测试位置" ("Status")) -> ()  [unwired: 11 in]
              }
              frame 56 {
                n181 = call "浮动通知.vi"("通知内容"="夹爪夹紧" ("Status")) -> ()  [unwired: 11 in]
              }
              frame 61 {
                n182 = call "浮动通知.vi"("通知内容"="测试完成夹爪松开" ("Status")) -> ()  [unwired: 11 in]
              }
              frame 62 {
                n183 = call "浮动通知.vi"("通知内容"="TOX电缸返程" ("Status")) -> ()  [unwired: 11 in]
              }
              frame 63 {
                n184 = call "浮动通知.vi"("通知内容"="请锁紧手柄" ("Status")) -> ()  [unwired: 11 in]
              }
              frame 100 {
                n185 = call "浮动通知.vi"("通知内容"="压紧气缸伸出！" ("Status")) -> ()  [unwired: 11 in]
              }
              frame 105 {
                n186 = call "浮动通知.vi"("通知内容"="压紧缸下降！" ("Status")) -> ()  [unwired: 11 in]
              }
              frame 120 {
                n187 = call "浮动通知.vi"("通知内容"="夹爪夹紧！" ("Status")) -> ()  [unwired: 11 in]
              }
              frame 130 {
                n188 = call "浮动通知.vi"("通知内容"="拉升磨合" ("Status")) -> ()  [unwired: 11 in]
              }
              frame 131 {
                n189 = call "浮动通知.vi"("通知内容"="压紧气缸升起" ("Status")) -> ()  [unwired: 11 in]
              }
              frame 161 {
                n190 = call "浮动通知.vi"("通知内容"="夹爪松开" ("Status")) -> ()  [unwired: 11 in]
                n191 = local write "STEP"("判定" ("STEP")) -> ()
              }
              frame 163 {
                n192 = call "浮动通知.vi"("通知内容"="请取记号笔" ("Status")) -> ()  [unwired: 11 in]
              }
              frame 999 {
                n193 = call "浮动通知.vi"("通知内容"="请启动！" ("Status")) -> ()  [unwired: 11 in]
              }
              frame 1000 {
              }
              frame 1002 {
              }
              frame 1024 {
                n194 = local write "STEP"("退出自动" ("STEP")) -> ()
              }
            }
            n195 = call "备用1.vi"() -> ("Status_Read"=w201:i16)  [unwired: 11 in]
            n196 = case shown="100" w201 {
              frame 0, Default {
              }
              frame 100 {
                n197 = local write "STEP"("判定" ("STEP")) -> ()
              }
              frame 4 {
                n198 = local write "STEP"("初始化" ("STEP")) -> ()
              }
              frame 5 {
                n199 = local read "拉压曲线"() -> (w205:cluster{dbl[], dbl[]}[])
                n200 = global read "判定参数.vi" "判定框"() -> (w207:T5)
                n201 = for {
                  tunnel: w205 -> [w210] mode=indexing
                  tunnel: [w209] -> w206 mode=indexing
                  tunnel: w207 -> [w208]
                  i -> [w211]
                  n202 = case shown="0" w211 {
                    tunnel: w210 -> [w212 _ _]
                    tunnel: [w212 w215 w225] -> w209
                    tunnel: w208 -> [_ w220 w226]
                    frame Default {
                    }
                    frame 0 {
                      n203 = Unbundle By Name(w220) -> ("位移.下限"=w219:dbl, "位移.上限"=w218:dbl, "拉力.下限"=w213:dbl, "拉力.上限"=w214:dbl)
                      n204 = Build Array(w218, w218, w219, w219, w218) -> (w217:dbl[])
                      n205 = Build Array(w213, w214, w214, w213, w213) -> (w216:dbl[])
                      n206 = Bundle(w217, w216) -> (w215:cluster{dbl[], dbl[]})  [unwired: 1 in]
                    }
                    frame 1 {
                      n207 = Unbundle By Name(w226) -> ("位移1.下限"=w230:dbl, "位移1.上限"=w229:dbl, "压力.上限"=w223:dbl, "压力.下限"=w224:dbl)
                      n208 = Negate(x=w224) -> (-x=w221:dbl)
                      n209 = Negate(x=w223) -> (-x=w222:dbl)
                      n210 = Build Array(w229, w229, w230, w230, w229) -> (w228:dbl[])
                      n211 = Build Array(w222, w221, w221, w222, w222) -> (w227:dbl[])
                      n212 = Bundle(w228, w227) -> (w225:cluster{dbl[], dbl[]})  [unwired: 1 in]
                    }
                  }
                }
                n213 = local write "拉压曲线"(w206) -> ()
              }
              frame 1 {
                n214 = global read "Global.vi" "传感器读数"() -> (w233:T7)
                n215 = Unbundle By Name(w233) -> ("电缸位移"=w232:sgl, "拉压力"=w231:sgl)
                n216 = control-ref of="拉压曲线"() -> (w235:refnum<vi>)
                n217 = call "曲线采集.vi"("曲线引用"=w235, "曲线索引"=2, "X"=w232, "Y"=w231) -> ()  [unwired: 10 in, 2 out]
              }
              frame 2 {
                n218 = global read "Global.vi" "传感器读数"() -> (w238:T7)
                n219 = Unbundle By Name(w238) -> ("电缸位移"=w237:sgl, "拉压力"=w236:sgl)
                n220 = control-ref of="拉压曲线"() -> (w240:refnum<vi>)
                n221 = call "曲线采集.vi"("曲线引用"=w240, "曲线索引"=3, "X"=w237, "Y"=w236) -> ()  [unwired: 10 in, 2 out]
              }
            }
          }
          frame "合格判定" {
            n222 = Wait (ms)(milliseconds to wait=u32 100 ("等待时间（毫秒）")) -> ()  [unwired: 1 out]
            n223 = local write "STEP"("等待" ("STEP")) -> ()
          }
          frame "报表" {
            n224 = stacked-sequence {
              seq-local: [_ w277 _ _] -> [_ _ w282 _]
              frame #0 {
                n225 = global write "Global.vi" "计时开始"(FALSE ("计时开始")) -> ()
                n226 = disable-structure shown="禁用" {
                  frame Disabled {
                    n227 = global read "Global.vi" "产品编号"() -> (w276:string)
                    n228 = call "Get_CODE_ID.vi"("CODE_MAIN"=w276) -> ("CODE_ID"=w275:string)  [unwired: 10 in]
                    n229 = global write "追溯Global.vi" "CODE_ID"(w275) -> ()
                  }
                  frame Enabled {
                  }
                }
              }
              frame #1 {
                n230 = global read "Global.vi" "产品编号"() -> (w278:string)
                n231 = call "Report.vi"("文件重命名"=TRUE, "文件名称"=w278, "检测结果"="判定结果") -> ("PRODUCT_VAULE"=w277:string)  [unwired: 7 in, 1 out]
              }
              frame #2 {
                n232 = global read "Global.vi" "联机模式"() -> (w281:enum16{"单机", "追溯"})
                n233 = case shown="\"追溯\"" w281 {
                  tunnel: w282 -> [_ w283]
                  frame "单机", Default {
                  }
                  frame "追溯" {
                    n234 = global read "Global.vi" "Result"() -> (w285:refnum<vi>)
                    n235 = property class="Tbl"(reference=w285) -> (reference out=w290:refnum<vi>, error out=w287:errorcluster, "Row Headers[]"=w288:string[])  [unwired: 1 in]
                    n236 = property class="Tbl"(reference=w290, error in=w287) -> (error out=w286:errorcluster, "Value"=w289:string[][])  [unwired: 1 out]
                    n237 = for {
                      tunnel: w289 -> [w297] mode=indexing
                      tunnel: w288 -> [w298] mode=indexing
                      tunnel: [w295] -> w284 mode=indexing if=w296
                      shift-right: [w294] -> _
                      shift-left: w286 -> [w294]
                      n238 = Build Array (concatenate)(w298, w297) -> (w295:string[])
                      n239 = Index Array(array=w297) -> (element=w299:string)  [unwired: 1 in]
                      n240 = case shown="\"\"" w299 {
                        tunnel: [TRUE FALSE] -> w296
                        frame Default {
                        }
                        frame "" {
                        }
                      }
                    }
                    n241 = global read "追溯Global.vi" "CODEMAIN_ID"() -> (w293:string)
                    n242 = global read "追溯Global.vi" "DEVICE_ID"() -> (w292:string)
                    n243 = global read "追溯Global.vi" "USER_ID"() -> (w291:string)
                    n244 = call "UPTEST.vi"("Result"=w284, "CODE_ID"=w293, "DEVICE_ID"=w292) -> ()  [unwired: 6 in, 1 out]
                    n245 = call "UPRESULT.vi"("DEVICE_ID"=w292, "USER_ID"=w291, "CODE_ID"=w293, "RESULT_VALUE"=w283) -> ()  [unwired: 11 in, 1 out]
                  }
                }
              }
              frame #3 {
                n246 = global read "检测结果.vi" "合格状态"() -> (w304:string)
                n247 = local write "STEP"("自动" ("STEP")) -> ()
                n248 = case shown="\"合格\"" w304 {
                  frame "假", Default {
                  }
                  frame "合格" {
                    n249 = global read "Global.vi" "合格数量"() -> (w307:i32)
                    n250 = Increment(x=w307) -> (x+1=w306:i32)
                    n251 = global write "Global.vi" "合格数量"(w306) -> ()
                  }
                }
                n252 = call "备用1.vi"("枚举"=enum16{"Read", "Write"}."Write", "Status_Write"=i16 1000) -> ()  [unwired: 9 in, 1 out]
              }
            }
          }
        }
        n253 = global read "Global.vi" "程序关闭"() -> (w26:bool)
      }
      n254 = while {
        shift-right: [w308] -> w23
        shift-left: w24 -> [w309]
        stop <- w310 stop-if-true
        n255 = event shown="[4] <产品>: 用户事件" {
          selector: w309 -> [_ _ _ _ _ _ _ _]
          dyn-events: [_ _ _ _ _ _ _ _] -> w308
          timeout: 200 -> [_ _ _ _ _ _ _ _]
          event Timeout {
            n256 = event-data() -> ()  [unwired: 1 in, 3 out]
            n257 = call "Obtain Broadcast Events for Registration.vi"() -> ("Already running?"=w312:bool)  [unwired: 9 in, 2 out]
            n258 = case shown="真" w312 {
              frame False {
                n259 = local write "STEP"("手动" ("STEP")) -> ()
              }
              frame True {
                n260 = call "错误代码.vi"() -> ("Status_Read"=w314:u32)  [unwired: 11 in]
                n261 = feedback #1() -> (w324:u32)  [unwired: 1 in]
                n262 = feedback-in #1(w314) -> ()
                n263 = case shown="0" w314 {
                  frame 0 {
                    n264 = global read "Global.vi" "报警图标"() -> (w325:refnum<vi>)
                    n265 = property class="Bool"(reference=w325, "Visible"=FALSE ("可见")) -> ()  [unwired: 1 in, 2 out]
                  }
                  frame 1, Default {
                    n266 = global read "Global.vi" "报警图标"() -> (w328:refnum<vi>)
                    n267 = property class="Bool"(reference=w328, "Visible"=TRUE ("可见")) -> ()  [unwired: 1 in, 2 out]
                  }
                }
                n268 = Greater Or Equal?(x=w314, y=i16 5000) -> (x >= y?=w322:bool)
                n269 = Less?(x=w314, y=i16 5200) -> (x < y?=w323:bool)
                n270 = Equal?(x=w314, y=w324) -> (x = y?=w321:bool)
                n271 = global read "Global.vi" "报警图标"() -> (w316:refnum<vi>)
                n272 = And(x=w322, y=w323) -> (x .and. y?=w315:bool)
                n273 = property class="Bool"(reference=w316, "Value"=w315) -> ()  [unwired: 1 in, 2 out]
                n274 = Bundle By Name(cluster=errorcluster {"status"=FALSE, "code"=0, "source"=""} ("错误常量"), "status"=w315, "code"=w314) -> (w320:errorcluster)
                n275 = case shown="假" w321 {
                  tunnel: w320 -> [w329 _]
                  frame False {
                    n276 = call "报警处理.vi"("错误常量"=w329) -> ()  [unwired: 9 in, 2 out]
                  }
                  frame True {
                  }
                }
              }
            }
          }
          event User Event {
            n277 = event-data() -> ("试验项目"=w330:T1)  [unwired: 1 in]
            "试验项目" <- w330
            n278 = disable-structure shown="禁用" {
              disable-tunnel: w330 -> [w331 _]
              frame Disabled {
                n279 = global read "A180648.vi" "检测结果"() -> (w334:string[][][])
                n280 = global read "Global.vi" "Result"() -> (w332:refnum<vi>)
                n281 = Index Array(array=w334, index (dim 0)=w331) -> (element=w333:string[][])  [unwired: 2 in]
                n282 = property class="Tbl"(reference=w332, "Value"=w333) -> ()  [unwired: 1 in, 2 out]
              }
              frame Enabled {
              }
            }
          }
          event "试验项目": Value Change {
            n283 = event-data() -> ("NewVal"=w335:T1)  [unwired: 1 in]
            n284 = disable-structure shown="禁用" {
              disable-tunnel: w335 -> [w339 _]
              frame Disabled {
                n285 = global read "A180648.vi" "检测结果"() -> (w338:string[][][])
                n286 = global read "Global.vi" "Result"() -> (w336:refnum<vi>)
                n287 = Index Array(array=w338, index (dim 0)=w339) -> (element=w337:string[][])  [unwired: 2 in]
                n288 = property class="Tbl"(reference=w336, "Value"=w337) -> ()  [unwired: 1 in, 2 out]
              }
              frame Enabled {
              }
            }
          }
          event "0°曲线", "侧铆曲线", "45°曲线", "拉压曲线", "功能试验", "逆向空载试验", "磨合": Scale Range Change {
            n289 = event-data() -> ("CtlRef"=w341:refnum<vi>)  [unwired: 1 in, 4 out]
            n290 = global read "Global.vi" "产品型号"() -> (w340:string)
            n291 = call "XY_conf.vi"("方式"=enum16{"写入", "读取"}."写入", "产品"=w340, "XY图引用"=w341) -> ()  [unwired: 4 in, 1 out]
          }
          event User Event {
            n292 = event-data() -> ("产品"=w345:string)  [unwired: 1 in]
            n293 = control-ref of="0°曲线"() -> (w344:refnum<vi>)
            n294 = control-ref of="拉压曲线"() -> (w347:refnum<vi>)
            n295 = control-ref of="45°曲线"() -> (w343:refnum<vi>)
            n296 = control-ref of="侧铆曲线"() -> (w349:refnum<vi>)
            n297 = control-ref of="力特性试验"() -> (w348:refnum<vi>)
            n298 = Build Array(w344, w347, w343, w349, w348) -> (w346:refnum<vi>[])
            n299 = for {
              tunnel: w346 -> [w351] mode=indexing
              tunnel: w345 -> [w350]
              n300 = call "XY_conf.vi"("方式"=enum16{"写入", "读取"}."读取", "产品"=w350, "XY图引用"=w351) -> ()  [unwired: 4 in, 1 out]
            }
          }
          event Panel Close {
            n301 = event-data() -> ()  [unwired: 1 in, 4 out]
            n302 = global write "Global.vi" "程序关闭"(TRUE ("程序关闭")) -> ()
          }
          event "0°曲线", "侧铆曲线", "45°曲线", "拉压曲线", "功能试验", "逆向空载试验", "磨合": Mouse Enter; "0°曲线", "侧铆曲线", "45°曲线", "拉压曲线", "功能试验", "逆向空载试验", "磨合": Mouse Leave; "0°曲线", "侧铆曲线", "45°曲线", "拉压曲线", "功能试验", "逆向空载试验": Cursor Move; "磨合": Mouse Move {
            n303 = event-data() -> ("CtlRef"=w355:refnum<vi>, "Type"=w354:T8)  [unwired: 1 in]
            n304 = disable-structure shown="禁用" {
              disable-tunnel: w355 -> [w358 _]
              disable-tunnel: w354 -> [w356 _]
              frame Disabled {
                n305 = call "CursorShow.vi"("nameShow"=TRUE, "Type"=w356, "Graph"=w358) -> ()  [unwired: 7 in, 2 out]
              }
              frame Enabled {
              }
            }
          }
          event "0°曲线", "侧铆曲线", "45°曲线", "拉压曲线", "功能试验", "逆向空载试验", "磨合": Mouse Down {
            n306 = event-data() -> ("CtlRef"=w361:refnum<vi>, "Coords"=w360:T9, "Type"=w359:T8)  [unwired: 1 in]
            n307 = disable-structure shown="禁用" {
              disable-tunnel: w361 -> [w366 _]
              disable-tunnel: w360 -> [w365 _]
              disable-tunnel: w359 -> [w363 _]
              frame Disabled {
                n308 = invoke class="XYGraph (严格)" method="Map Coords To XY"(reference=w366, "Coords"=w365) -> (reference out=w364:refnum<vi>, "XY"=w362:cluster{"X":dbl, "Y":dbl})  [unwired: 5 in, 5 out]
                n309 = call "CursorShow.vi"("游标.游标位置"=w362, "Type"=w363, "Graph"=w364) -> ()  [unwired: 7 in, 2 out]
              }
              frame Enabled {
              }
            }
          }
        }
        n310 = global read "Global.vi" "程序关闭"() -> (w310:bool)
      }
    }
  }
  n311 = Unregister For Events(event registration refnum=w5) -> ()  [unwired: 1 in, 1 out]
